vi "ATE_NS_DL_cal2.vi"() -> ()   [LabVIEW 2009]
doc: "Use this template to build a producer/consumer design pattern with events to produce queue items. Use this design pattern instead of the User Interface Event Handler pattern for user interfaces when you want to execute code asynchronously in response to an event without slowing the user interface responsiveness."
uses:
  Rvp8PowerData.ctl
  <vilib>/Analysis/NI_AALBase.lvlib
panel:
  in  "70 dB Attn":i32=70 min=0 max=70 step=10
  in  "READY":bool
  out "Instructions":string="Noise Source Dummy Load calibration vi\n\n1 - Disable or turn off transmitter\n2 - Stow Antenna (point vertically)\n3 - Turn off all florescnt lights\n3 - Start the labview program by clicking the Run arrow\n     (left most button under  drop down menues)\n     start cycle time about 35 seconds\n4 - Wait for the red 'BUSY' light to change to green 'READY'\n     All the control buttons on the control panel are avtive.\n5 - Calibrate with the red  'Calibrate' button\n      calibration cycle time is about ? minutes\n6 - Exit the program with the red 'EXIT' button\n      exit cycle time about 20 seconds\n\nHints:\nWait for the green 'READY' light before clicking buttons\nAll the status leds on the 'Status' tab should be green during a calibration. "
  in  "Configuration 1":bool
  out "Cal Output File":path
  out "Cal file name":string
  in  "Cal data directory":string="/home/operator/ate/data/rvp8_cal"
  in  "Set SigGen":bool
  in  "Initialize":bool
  in  "70 dB":bool
  in  "121 dB":bool
  in  "Switches":bool
  in  "Calibrate":bool
  in  "Stop":bool
  in  "ATE TABS":enum32{"Status", "Controls"}(tab)=enum."Controls"
  out "ATE Switch Status":T1
  out "RVP8 Power":T2 {"time" format="%<%H:%M:%S\n%Y/%m/%d>T"}
  out "121dB\nAttenuators":bool[](array[boolean])
  out "121 Verified":bool
  out "Inside Noise Box":bool
  in  "WG3 MS":bool
  in  "WG3 T":bool
  out "WG3":bool
  in  "WG2 MS":bool
  in  "WG2 T":bool
  out "WG2":bool
  in  "WG1 MS":bool
  in  "WG1 T":bool
  out "WG1":bool
  in  "WG5 ANT":bool
  in  "WG5 DL":bool
  out "WG5":bool
  in  "WG4 ANT":bool
  in  "WG4 DL":bool
  out "WG4":bool
  in  "ATE Switches":T3={"Reversing Switch"=enum."Normal Function", "IO Switch #1 Input"=enum."NONE", "IO Switch #1 Output"=enum."NONE", "IO Switch #2 Input"=enum."NONE", "IO Switch #2 Output"=enum."NONE", "Signal Out Input"=enum."NONE", "Signal Out Output"=enum."NONE", "Signal Source Input"=enum."NONE", "Signal Source Output"=enum."NONE", "Power Meter Switch Input"=enum."NONE", "Pouer Meter Switch Output"=enum."NONE", "Amplifier Switch"=enum."Include Amp"}
  in  "DataSource":bool=TRUE
  in  "Measurements":i32=10
  in  "121 dB Atten":i32 min=0 max=121 step=1
  in  "NoiseSource":bool
  in  "NS_on/off":bool
  in  "Wave Guide Termination":bool
  out "P-State":string
  out "C-State":string
  in  "BUSY":bool
  # "ATE NS DL Program"
  # "1 dB"
  # "2 dB"
  # "4 dB"
  # "4 dB"
  # "10 dB"
  # "20 dB"
  # "40 dB"
  # "40 dB"
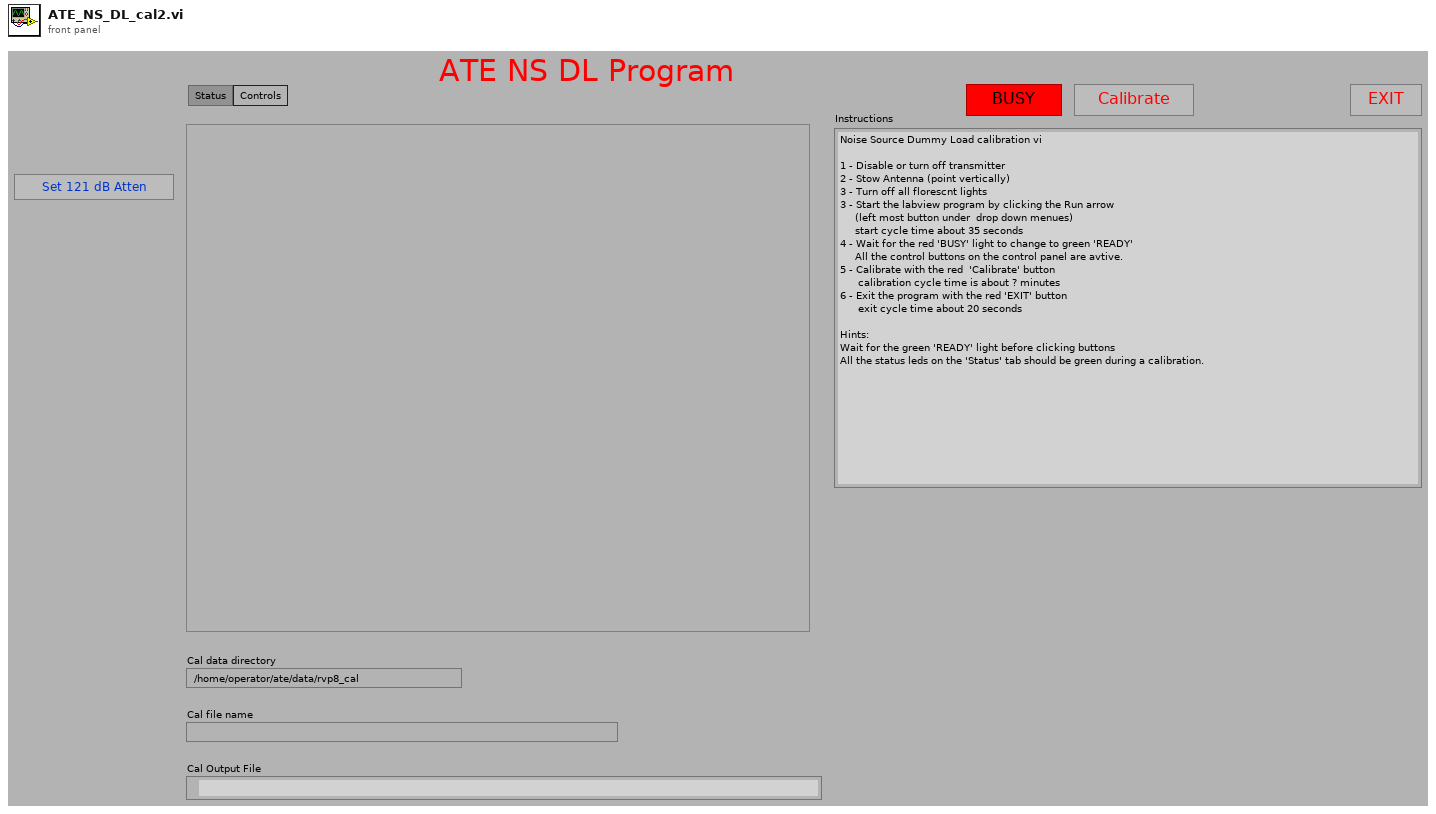
[diagram p1: front panel]
types:
  T1 = cluster{"Reversing Switch ":bool, "IO Switch #1":bool, "IO Switch #2":bool, "Signal Out":bool, "Signal Source":bool, "Power Meter":bool, "Amp By Pass":bool}
  T2 = typedef "Rvp8PowerData.ctl" = cluster{"success":bool, "time":dbl, "el":dbl, "az":dbl, "dbm0":dbl, "dbm1":dbl, "dbmHc":dbl, "dbmHx":dbl, "dbmVc":dbl, "dbmVx":dbl}
  T3 = cluster{"Reversing Switch":enum16{"Normal Function", "Reversing Function"}, "IO Switch #1 Input":enum16{"NONE", "AHR (J2)", "Splitter", "Signal Out Switch (S3)", "Reversing Switch"}, "IO Switch #1 Output":enum16{"NONE", "AHR (J2)", "Delay Device (S4)", "Power Meter Switch (S5)", "Reversing Switch"}, "IO Switch #2 Input":enum16{"NONE", "AVR (J3)", "Splitter", "Signal Out Switch (S3)", " 2W Term (TM1)", "Reversing Switch"}, "IO Switch #2 Output":enum16{"NONE", "AVR (J3)", "Signal Out Switch (S3)", "Power Meter Switch (S5)", "Reversing Switch", "2W Term (TM1)"}, "Signal Out Input":enum16{"NONE", "Amp Bypass Switch (S6)", "IO Switch #1 (S1)", "IO Switch #2 (S2)", "2W Term (TM3)"}, "Signal Out Output":enum16{"NONE", "2 Watt Term (TM3)", "Splitter", "Power Meter Switch (S5)"}, "Signal Source Input":enum16{"NONE", "Delay Device", "Signal Generator (J7)", "Inside Noise Box NF (J5)", "2W Term (TM3)"}, "Signal Source Output":enum16{"NONE", "Amp Bypass Switch", "Test Pulse Generator", "Power Meter Switch (S5)"}, "Power Meter Switch Input":enum16{"NONE", "IO Switch #1 (S1)", "Signal Source Switch (S4)", "Signal Out Switch (S3)", "IO Switch #2 (S2)", "TXH-TXV Switch (J8)"}, "Pouer Meter Switch Output":enum16{"NONE", "Power Meter (J6)"}, "Amplifier Switch":enum16{"Bypass Amp", "Include Amp"}}
  T4 = cluster{"Frequency (GHz)":dbl, "RF Power (dBm)":dbl, "RF ON/OFF":bool}
  T5 = enum16{"open", "replace", "create", "open or create", "replace or create", "replace or create with confirmation"}
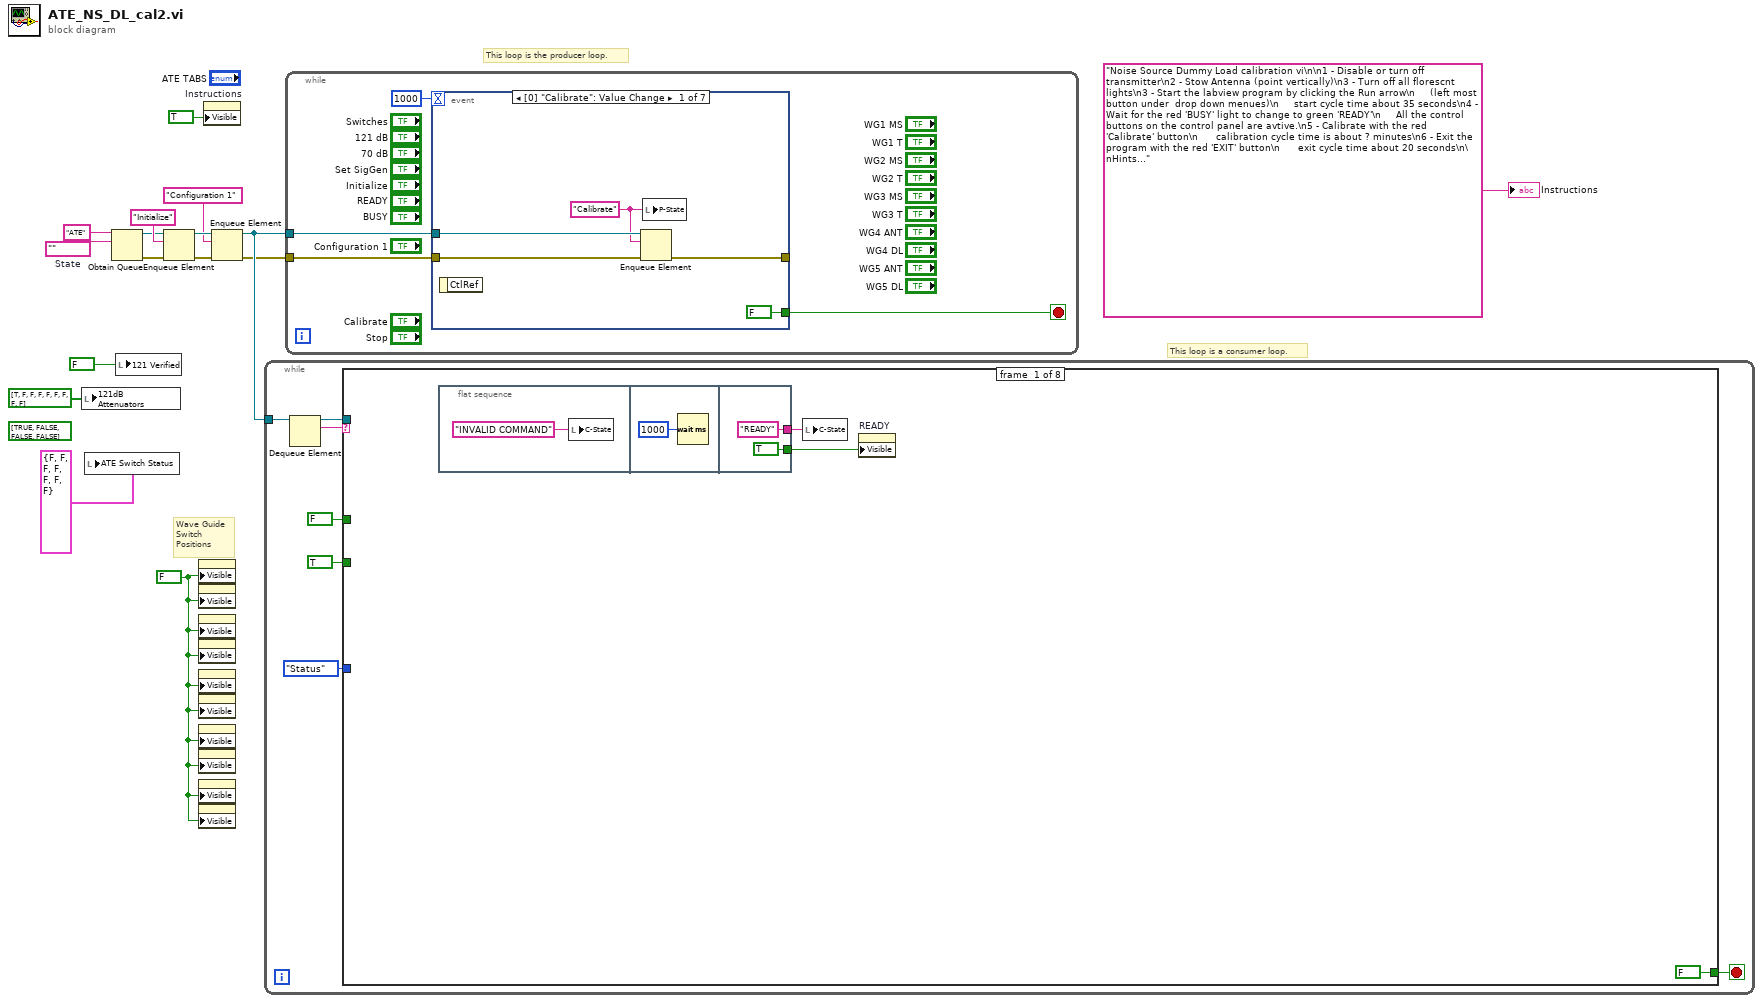
[diagram p0: block diagram]
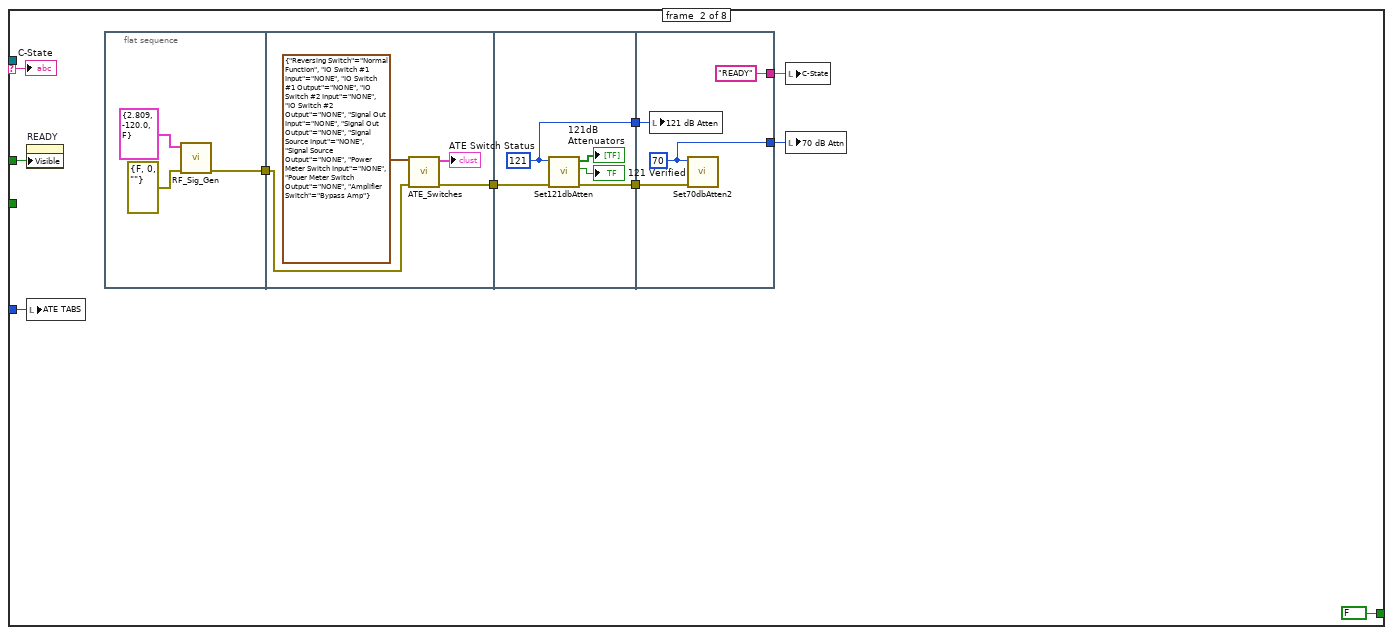
[diagram p2: hidden frame]
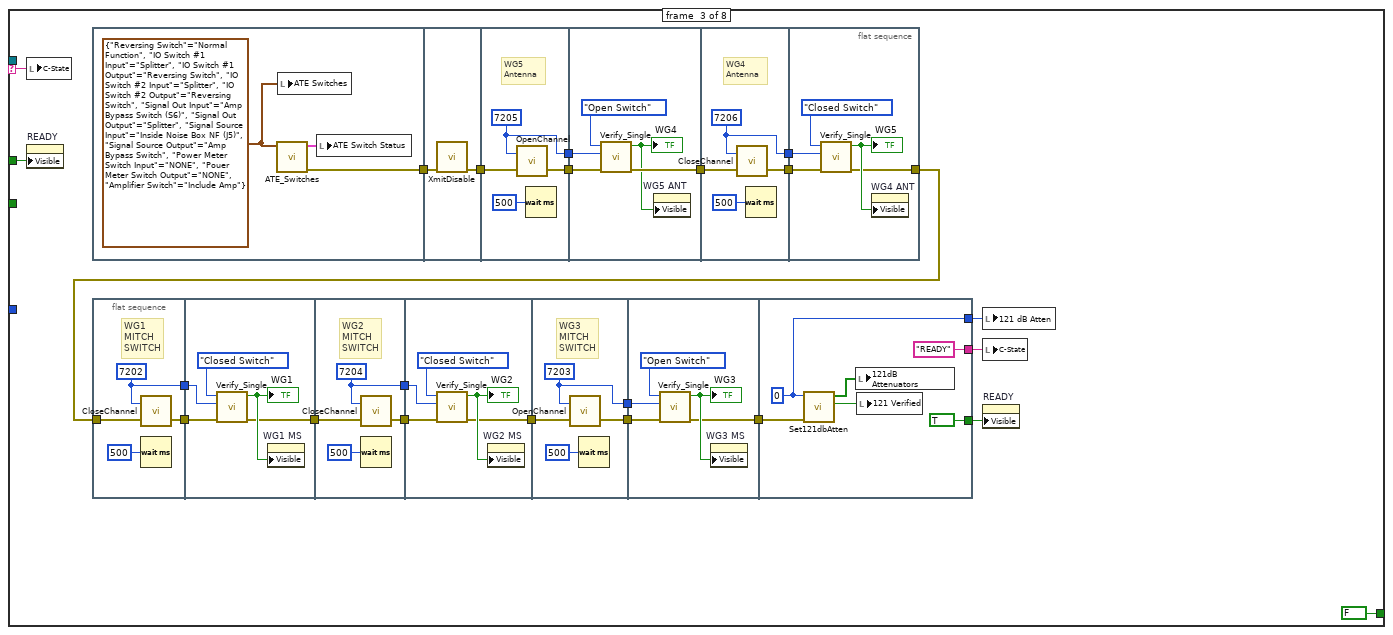
[diagram p3: hidden frame]
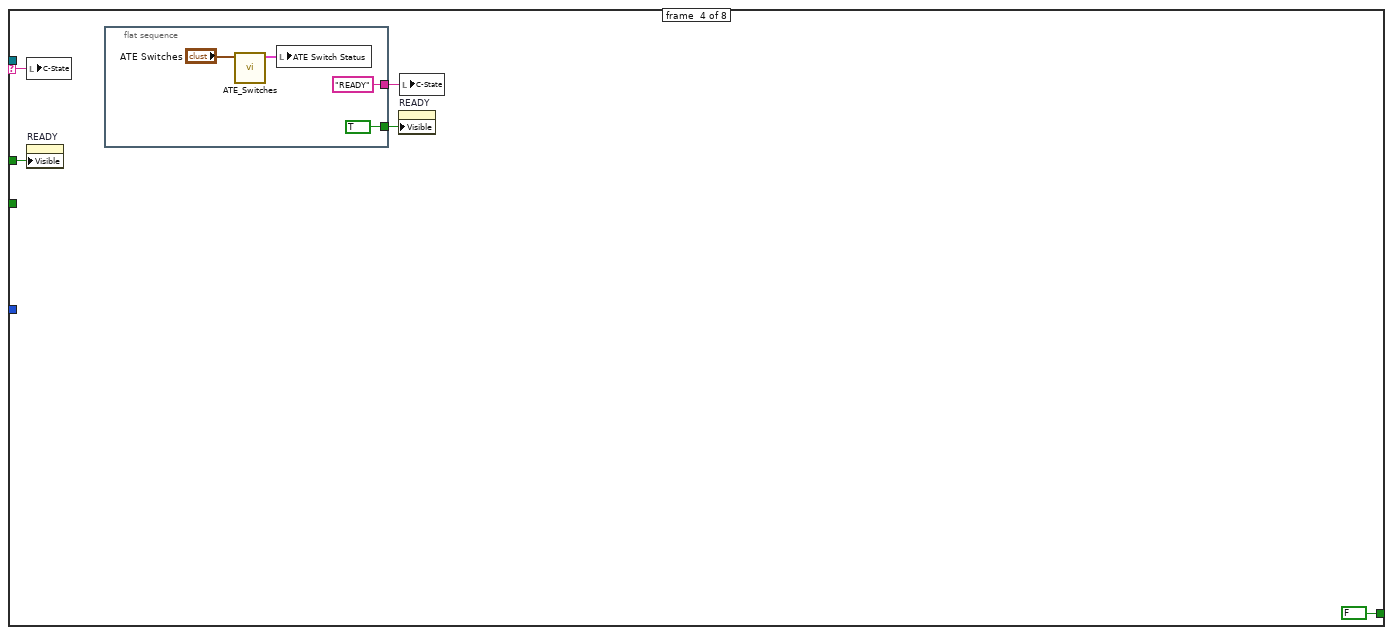
[diagram p4: hidden frame]
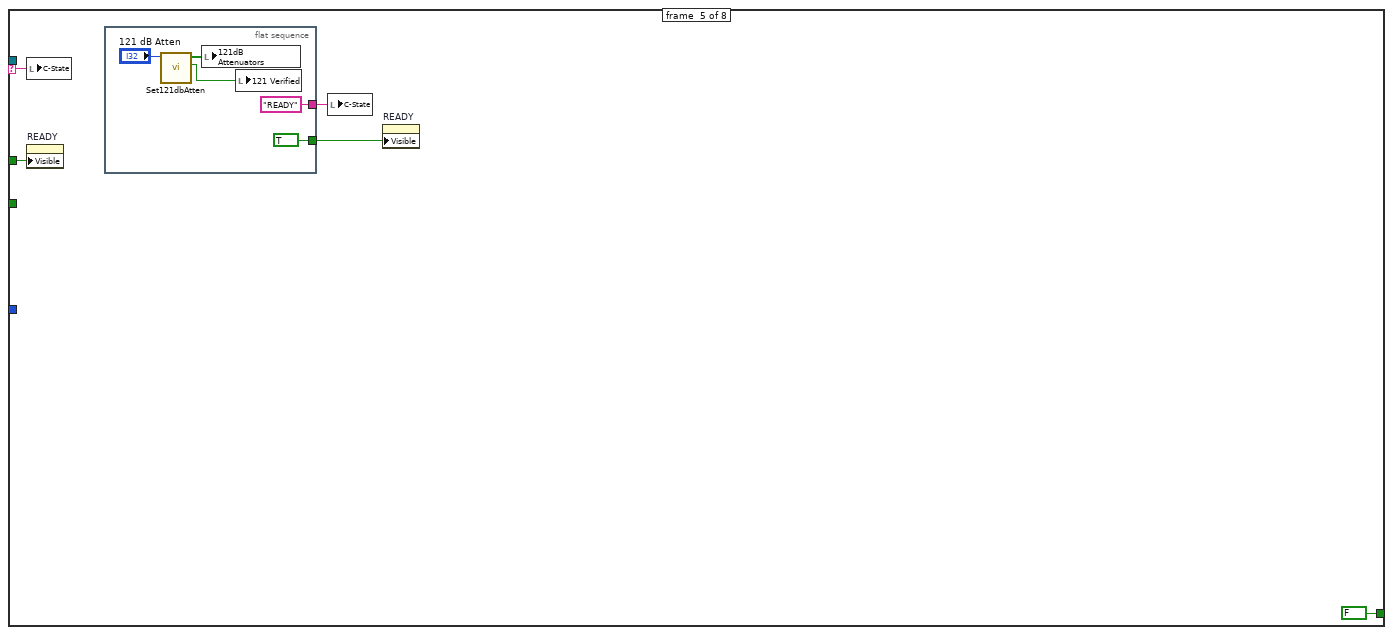
[diagram p5: hidden frame]
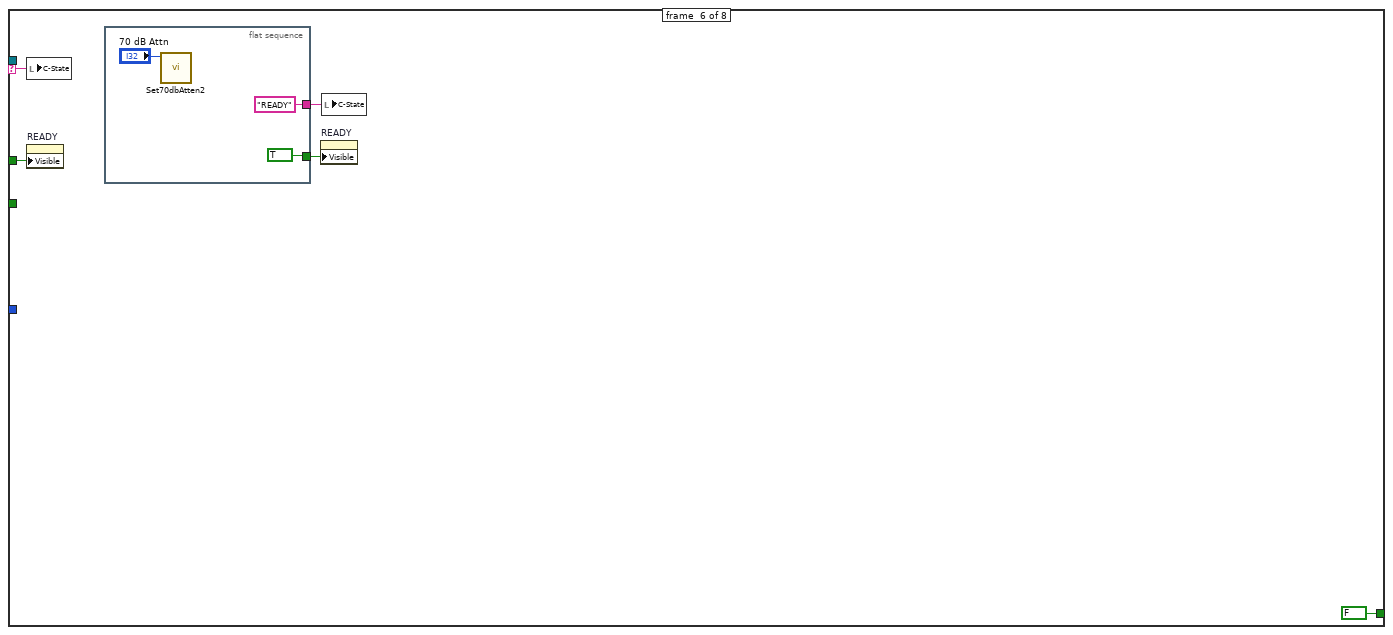
[diagram p6: hidden frame]
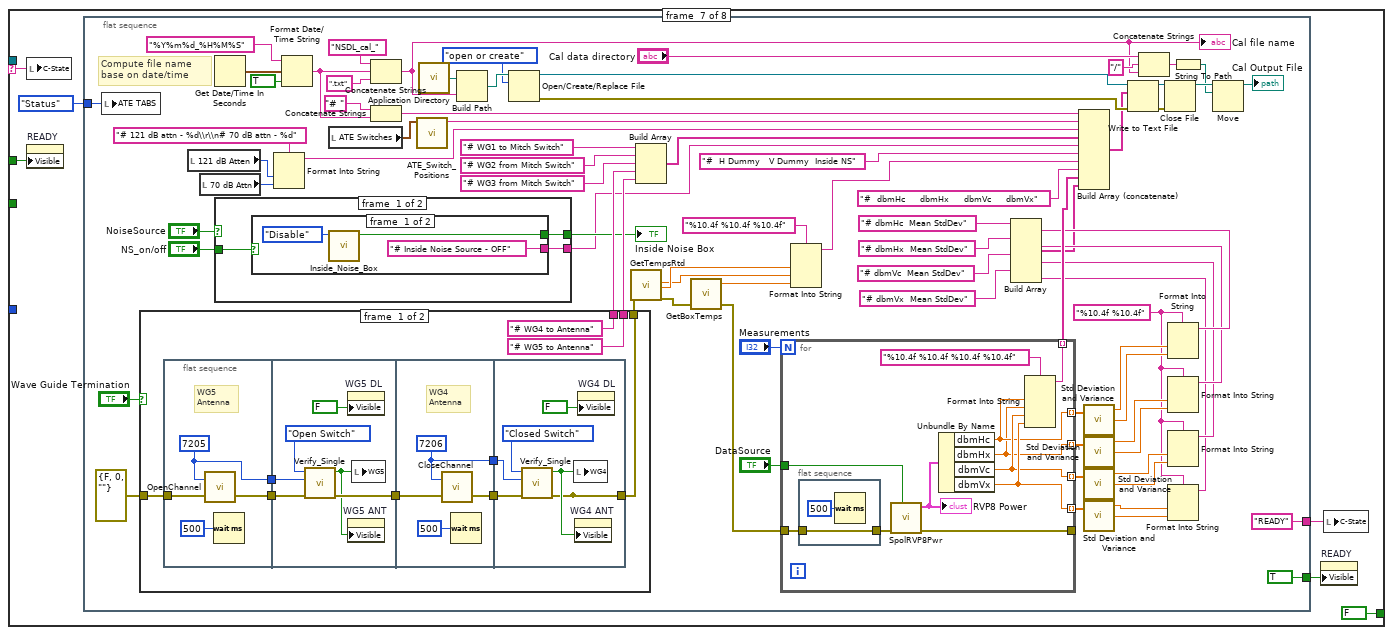
[diagram p7: hidden frame]
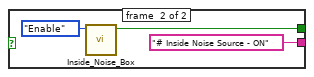
[diagram p8: hidden frame]
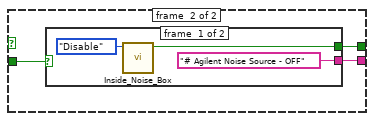
[diagram p9: hidden frame]
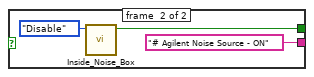
[diagram p10: hidden frame]
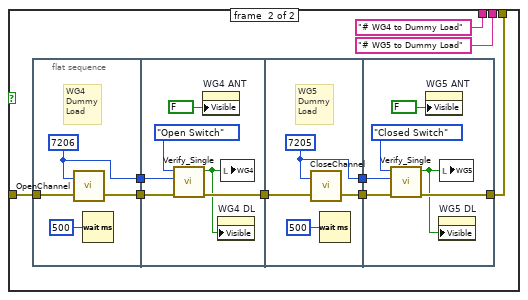
[diagram p11: hidden frame]
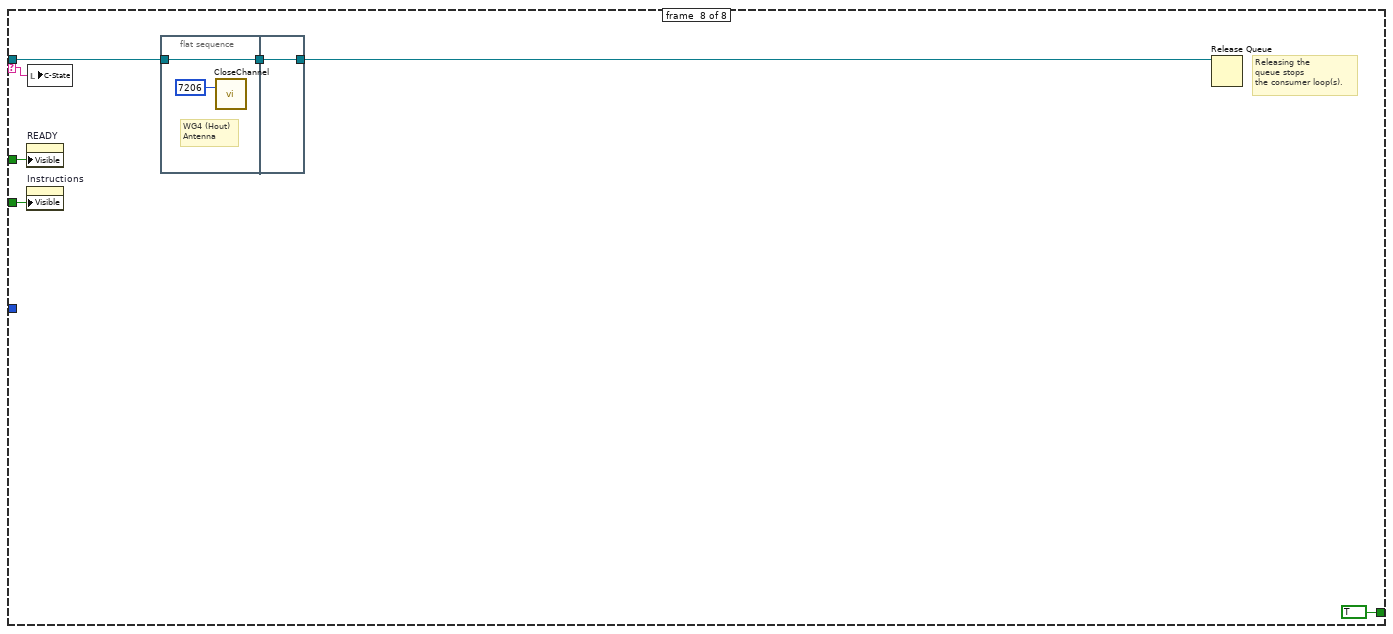
[diagram p12: hidden frame]
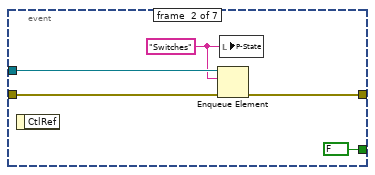
[diagram p13: hidden frame]
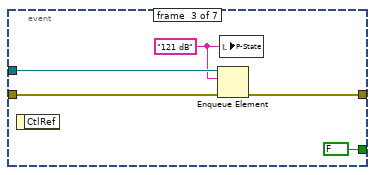
[diagram p14: hidden frame]
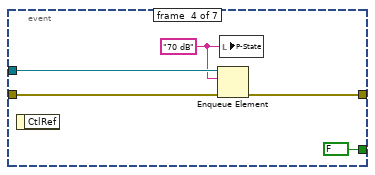
[diagram p15: hidden frame]
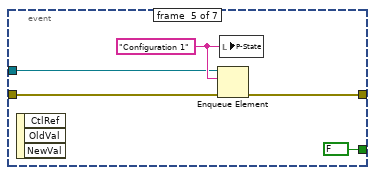
[diagram p16: hidden frame]
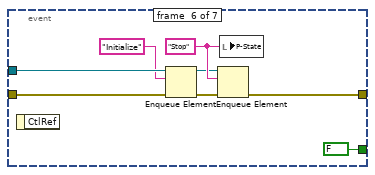
[diagram p17: hidden frame]
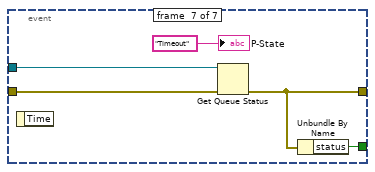
[diagram p18: hidden frame]
diagram:
  w5 = FALSE ("Visible")
  (unwired) bool[] [TRUE, FALSE, FALSE, FALSE] ("70dB\nAttenuators")
  w16 = ""  # State
  # "Wave Guide\nSwitch\nPositions"
  # "This loop is the producer loop."
  # "This loop is a consumer loop."
  n1 = local write "121dB\nAttenuators"(bool[] [TRUE, FALSE, FALSE, FALSE, FALSE, FALSE, FALSE, FALSE, FALSE] ("121dB\nAttenuators")) -> ()
  n2 = local write "ATE Switch Status"(T1 {"Reversing Switch "=FALSE, "IO Switch #1"=FALSE, "IO Switch #2"=FALSE, "Signal Out"=FALSE, "Signal Source"=FALSE, "Power Meter"=FALSE, "Amp By Pass"=FALSE} ("ATE Switch Status")) -> ()
  n3 = Obtain Queue(name (unnamed)="ATE", element data type=w16) -> (queue out=w13:refnum<queue>, error out=w12:errorcluster)  [unwired: 3 in, 1 out]
  n4 = local write "121 Verified"(FALSE ("70 Verfied")) -> ()
  n5 = Enqueue Element(queue=w13, element="Initialize", error in (no error)=w12) -> (queue out=w6:refnum<queue>, error out=w3:errorcluster)  [unwired: 1 in, 1 out]
  n6 = property on="WG1 MS" class="Bool"("Visible"=w5) -> ()  [unwired: 2 in, 2 out]
  n7 = property on="WG1 T" class="Bool"("Visible"=w5) -> ()  [unwired: 2 in, 2 out]
  n8 = property on="WG2 MS" class="Bool"("Visible"=w5) -> ()  [unwired: 2 in, 2 out]
  n9 = property on="WG2 T" class="Bool"("Visible"=w5) -> ()  [unwired: 2 in, 2 out]
  n10 = property on="WG3 MS" class="Bool"("Visible"=w5) -> ()  [unwired: 2 in, 2 out]
  n11 = property on="WG3 T" class="Bool"("Visible"=w5) -> ()  [unwired: 2 in, 2 out]
  n12 = property on="WG4 ANT" class="Bool"("Visible"=w5) -> ()  [unwired: 2 in, 2 out]
  n13 = property on="WG4 DL" class="Bool"("Visible"=w5) -> ()  [unwired: 2 in, 2 out]
  n14 = property on="WG5 ANT" class="Bool"("Visible"=w5) -> ()  [unwired: 2 in, 2 out]
  n15 = property on="WG5 DL" class="Bool"("Visible"=w5) -> ()  [unwired: 2 in, 2 out]
  n16 = property on="Instructions" class="Str"("Visible"=TRUE) -> ()  [unwired: 2 in, 2 out]
  n17 = Enqueue Element(queue=w6, element="Configuration 1", error in (no error)=w3) -> (queue out=w4:refnum<queue>, error out=w2:errorcluster)  [unwired: 1 in, 1 out]
  n18 = while {
    tunnel: w4 -> [w23]
    stop <- w20 stop-if-true
    n19 = Dequeue Element(queue=w23) -> (queue out=w21:refnum<queue>, element=w22:string)  [unwired: 2 in, 2 out]
    n20 = case shown="\"Calibrate\"" w22 {
      selector: w22 -> [_ w39 w77 w140 w148 w158 w167 w342]
      tunnel: w21 -> [_ _ _ _ _ _ _ w339]
      tunnel: [FALSE FALSE FALSE FALSE FALSE FALSE FALSE TRUE] -> w20
      tunnel: FALSE ("Visible") -> [_ w32 w76 w137 w146 w156 w165 w341]
      tunnel: TRUE ("Visible") -> [_ _ _ _ _ _ _ w340]
      tunnel: enum32{"Status", "Controls"}."Status" ("ATE TABS") -> [_ w31 _ _ _ _ _ _]
      frame #0 {
        n21 = flat-sequence {
          tunnel: ["READY" ("element")] -> w25
          tunnel: [TRUE ("Visible")] -> w24
          frame #0 {
            n22 = local write "C-State"("INVALID COMMAND" ("C-State")) -> ()
          }
          frame #1 {
            n23 = Wait (ms)(milliseconds to wait=u32 1000) -> ()  [unwired: 1 out]
          }
          frame #2 {
          }
        }
        n24 = local write "C-State"(w25) -> ()
        n25 = property on="READY" class="Bool"("Visible"=w24) -> ()  [unwired: 2 in, 2 out]
      }
      frame #1 {
        n26 = property on="READY" class="Bool"("Visible"=w32) -> ()  [unwired: 2 in, 2 out]
        n27 = local write "ATE TABS"(w31) -> ()
        n28 = flat-sequence {
          tunnel: [w41] -> w33
          tunnel: [w45] -> w36
          tunnel: w33 -> [w46]
          tunnel: w36 -> [w51]
          tunnel: [w50] -> w37
          tunnel: [w49] -> w35
          tunnel: ["READY" ("element")] -> w38
          tunnel: w37 -> [w56]
          tunnel: w35 -> [w54]
          tunnel: [w53] -> w34
          frame #0 {
            n29 = call "RF_Sig_Gen.vi"("error in"=errorcluster {"status"=FALSE, "code"=0, "source"=""}, "Signal Generator Control"=T4 {"Frequency (GHz)"=2.809, "RF Power (dBm)"=-120.0, "RF ON/OFF"=FALSE}) -> ("Sig Gen Errors"=w41:errorcluster)  [unwired: 8 in, 1 out]
          }
          frame #1 {
            n30 = call "ATE_Switches.vi"("error in"=w46, "ATE Switches"=T3 {"Reversing Switch"=enum."Normal Function", "IO Switch #1 Input"=enum."NONE", "IO Switch #1 Output"=enum."NONE", "IO Switch #2 Input"=enum."NONE", "IO Switch #2 Output"=enum."NONE", "Signal Out Input"=enum."NONE", "Signal Out Output"=enum."NONE", "Signal Source Input"=enum."NONE", "Signal Source Output"=enum."NONE", "Power Meter Switch Input"=enum."NONE", "Pouer Meter Switch Output"=enum."NONE", "Amplifier Switch"=enum."Bypass Amp"}) -> ("Switch Errors"=w45:errorcluster, "ATE Switch Status"=→"ATE Switch Status":T1)  [unwired: 8 in]
          }
          frame #2 {
            w49 = 121 ("Attenuation (dB)")
            n31 = call "Set121dbAtten.vi"("error in (no error)"=w51, "Attenuation (dB)"=w49) -> ("error out"=w50:errorcluster, "Verfied"=→"121 Verified":bool, "Active Attenuators"=→"121dB\nAttenuators":bool[])  [unwired: 7 in]
          }
          frame #3 {
            w53 = 70 ("Attenuation (dB)")
            n32 = local write "121 dB Atten"(w54) -> ()
            n33 = call "Set70dbAtten2.vi"("error in (no error)"=w56, "Attenuation (dB)"=w53) -> ()  [unwired: 7 in, 3 out]
          }
        }
        n34 = local write "C-State"(w38) -> ()
        n35 = local write "70 dB Attn"(w34) -> ()
        "C-State" <- w39
      }
      frame #2 {
        n36 = local write "C-State"(w77) -> ()
        n37 = property on="READY" class="Bool"("Visible"=w76) -> ()  [unwired: 2 in, 2 out]
        n38 = flat-sequence {
          tunnel: [w115] -> w78
          tunnel: w78 -> [w117]
          tunnel: [w116] -> w75
          tunnel: w75 -> [w121]
          tunnel: [w120] -> w72
          tunnel: [w119] -> w71
          tunnel: [w123] -> w74
          tunnel: w72 -> [w125]
          tunnel: w71 -> [w124]
          tunnel: [w128] -> w73
          tunnel: w74 -> [w130]
          tunnel: [w127] -> w59
          tunnel: w73 -> [w134]
          tunnel: w59 -> [w133]
          tunnel: [w131] -> w58
          frame #0 {
            w113 = T3 {"Reversing Switch"=enum."Normal Function", "IO Switch #1 Input"=enum."Splitter", "IO Switch #1 Output"=enum."Reversing Switch", "IO Switch #2 Input"=enum."Splitter", "IO Switch #2 Output"=enum."Reversing Switch", "Signal Out Input"=enum."Amp Bypass Switch (S6)", "Signal Out Output"=enum."Splitter", "Signal Source Input"=enum."Inside Noise Box NF (J5)", "Signal Source Output"=enum."Amp Bypass Switch", "Power Meter Switch Input"=enum."NONE", "Pouer Meter Switch Output"=enum."NONE", "Amplifier Switch"=enum."Include Amp"} ("ATE Switches")
            n39 = call "ATE_Switches.vi"("ATE Switches"=w113) -> ("Switch Errors"=w115:errorcluster, "ATE Switch Status"=w114:T1)  [unwired: 9 in]
            n40 = local write "ATE Switches"(w113) -> ()
            n41 = local write "ATE Switch Status"(w114) -> ()
          }
          frame #1 {
            n42 = call "XmitDisable.vi"("error in (no error)"=w117) -> ("error out"=w116:errorcluster)  [unwired: 1 in, 5 out]
          }
          frame #2 {
            w119 = 7205
            # "WG5\nAntenna"
            n43 = call "OpenChannel.vi"("error in (no error)"=w121, "Channel ID"=w119) -> ("error out"=w120:errorcluster)  [unwired: 1 in]
            n44 = Wait (ms)(milliseconds to wait=u32 500) -> ()  [unwired: 1 out]
          }
          frame #3 {
            n45 = call "Verify_Single.vi"("error in"=w125, "Switch ID"=w124, "Switch Functin"=enum16{"Open Switch", "Closed Switch"}."Open Switch") -> ("Error out"=w123:errorcluster, "Verfied"=w122:bool)  [unwired: 7 in]
            "WG4" <- w122
            n46 = property on="WG5 ANT" class="Bool"("Visible"=w122) -> ()  [unwired: 2 in, 2 out]
          }
          frame #4 {
            w127 = 7206
            # "WG4\nAntenna"
            n47 = call "CloseChannel.vi"("error in (no error)"=w130, "Channel ID"=w127) -> ("error out"=w128:errorcluster)  [unwired: 1 in]
            n48 = Wait (ms)(milliseconds to wait=u32 500) -> ()  [unwired: 1 out]
          }
          frame #5 {
            n49 = call "Verify_Single.vi"("error in"=w134, "Switch ID"=w133, "Switch Functin"=enum16{"Open Switch", "Closed Switch"}."Closed Switch") -> ("Error out"=w131:errorcluster, "Verfied"=w132:bool)  [unwired: 7 in]
            "WG5" <- w132
            n50 = property on="WG4 ANT" class="Bool"("Visible"=w132) -> ()  [unwired: 2 in, 2 out]
          }
        }
        n51 = flat-sequence {
          tunnel: [w82] -> w70
          tunnel: [w81] -> w67
          tunnel: w58 -> [w80]
          tunnel: w70 -> [w87]
          tunnel: [w85] -> w69
          tunnel: w67 -> [w84]
          tunnel: w69 -> [w91]
          tunnel: [w90] -> w68
          tunnel: [w89] -> w66
          tunnel: w68 -> [w96]
          tunnel: w66 -> [w95]
          tunnel: [w93] -> w65
          tunnel: w65 -> [w100]
          tunnel: [w99] -> w64
          tunnel: [w98] -> w63
          tunnel: w64 -> [w104]
          tunnel: w63 -> [w105]
          tunnel: [w102] -> w62
          tunnel: w62 -> [w108]
          tunnel: [TRUE ("Visible")] -> w61
          tunnel: ["READY" ("element")] -> w60
          tunnel: [w107] -> w57
          frame #0 {
            w81 = 7202
            # "WG1\nMITCH\nSWITCH"
            n52 = call "CloseChannel.vi"("error in (no error)"=w80, "Channel ID"=w81) -> ("error out"=w82:errorcluster)  [unwired: 1 in]
            n53 = Wait (ms)(milliseconds to wait=u32 500) -> ()  [unwired: 1 out]
          }
          frame #1 {
            n54 = call "Verify_Single.vi"("error in"=w87, "Switch ID"=w84, "Switch Functin"=enum16{"Open Switch", "Closed Switch"}."Closed Switch") -> ("Error out"=w85:errorcluster, "Verfied"=w86:bool)  [unwired: 7 in]
            "WG1" <- w86
            n55 = property on="WG1 MS" class="Bool"("Visible"=w86) -> ()  [unwired: 2 in, 2 out]
          }
          frame #2 {
            w89 = 7204
            # "WG2\nMITCH\nSWITCH"
            n56 = call "CloseChannel.vi"("error in (no error)"=w91, "Channel ID"=w89) -> ("error out"=w90:errorcluster)  [unwired: 1 in]
            n57 = Wait (ms)(milliseconds to wait=u32 500) -> ()  [unwired: 1 out]
          }
          frame #3 {
            n58 = call "Verify_Single.vi"("error in"=w96, "Switch ID"=w95, "Switch Functin"=enum16{"Open Switch", "Closed Switch"}."Closed Switch") -> ("Error out"=w93:errorcluster, "Verfied"=w94:bool)  [unwired: 7 in]
            "WG2" <- w94
            n59 = property on="WG2 MS" class="Bool"("Visible"=w94) -> ()  [unwired: 2 in, 2 out]
          }
          frame #4 {
            w99 = 7203
            # "WG3\nMITCH\nSWITCH"
            n60 = call "OpenChannel.vi"("error in (no error)"=w100, "Channel ID"=w99) -> ("error out"=w98:errorcluster)  [unwired: 1 in]
            n61 = Wait (ms)(milliseconds to wait=u32 500) -> ()  [unwired: 1 out]
          }
          frame #5 {
            n62 = call "Verify_Single.vi"("error in"=w105, "Switch ID"=w104, "Switch Functin"=enum16{"Open Switch", "Closed Switch"}."Open Switch") -> ("Error out"=w102:errorcluster, "Verfied"=w103:bool)  [unwired: 7 in]
            "WG3" <- w103
            n63 = property on="WG3 MS" class="Bool"("Visible"=w103) -> ()  [unwired: 2 in, 2 out]
          }
          frame #6 {
            w107 = 0 ("Attenuation (dB)")
            n64 = call "Set121dbAtten.vi"("error in (no error)"=w108, "Attenuation (dB)"=w107) -> ("Verfied"=w109:bool, "Active Attenuators"=w110:bool[])  [unwired: 7 in, 1 out]
            n65 = local write "121dB\nAttenuators"(w110) -> ()
            n66 = local write "121 Verified"(w109) -> ()
          }
        }
        n67 = local write "121 dB Atten"(w57) -> ()
        n68 = local write "C-State"(w60) -> ()
        n69 = property on="READY" class="Bool"("Visible"=w61) -> ()  [unwired: 2 in, 2 out]
      }
      frame #3 {
        n70 = local write "C-State"(w140) -> ()
        n71 = property on="READY" class="Bool"("Visible"=w137) -> ()  [unwired: 2 in, 2 out]
        n72 = flat-sequence {
          tunnel: ["READY" ("element")] -> w138
          tunnel: [TRUE ("Visible")] -> w136
          frame #0 {
            n73 = call "ATE_Switches.vi"("ATE Switches"="ATE Switches") -> ("ATE Switch Status"=w143:T1)  [unwired: 9 in, 1 out]
            n74 = local write "ATE Switch Status"(w143) -> ()
          }
        }
        n75 = property on="READY" class="Bool"("Visible"=w136) -> ()  [unwired: 2 in, 2 out]
        n76 = local write "C-State"(w138) -> ()
      }
      frame #4 {
        n77 = local write "C-State"(w148) -> ()
        n78 = property on="READY" class="Bool"("Visible"=w146) -> ()  [unwired: 2 in, 2 out]
        n79 = flat-sequence {
          tunnel: ["READY" ("element")] -> w147
          tunnel: [TRUE ("Visible")] -> w145
          frame #0 {
            n80 = call "Set121dbAtten.vi"("Attenuation (dB)"="121 dB Atten") -> ("Verfied"=w151:bool, "Active Attenuators"=w153:bool[])  [unwired: 8 in, 1 out]
            n81 = local write "121dB\nAttenuators"(w153) -> ()
            n82 = local write "121 Verified"(w151) -> ()
          }
        }
        n83 = local write "C-State"(w147) -> ()
        n84 = property on="READY" class="Bool"("Visible"=w145) -> ()  [unwired: 2 in, 2 out]
      }
      frame #5 {
        n85 = local write "C-State"(w158) -> ()
        n86 = property on="READY" class="Bool"("Visible"=w156) -> ()  [unwired: 2 in, 2 out]
        n87 = flat-sequence {
          tunnel: ["READY" ("element")] -> w157
          tunnel: [TRUE ("Visible")] -> w155
          frame #0 {
            n88 = call "Set70dbAtten2.vi"("Attenuation (dB)"="70 dB Attn") -> ()  [unwired: 8 in, 3 out]
          }
        }
        n89 = property on="READY" class="Bool"("Visible"=w155) -> ()  [unwired: 2 in, 2 out]
        n90 = local write "C-State"(w157) -> ()
      }
      frame #6 {
        n91 = local write "C-State"(w167) -> ()
        n92 = property on="READY" class="Bool"("Visible"=w165) -> ()  [unwired: 2 in, 2 out]
        n93 = flat-sequence {
          tunnel: ["READY" ("element")] -> w166
          tunnel: [TRUE ("Visible")] -> w164
          tunnel: enum32{"Status", "Controls"}."Status" ("ATE TABS") -> [w215]
          frame #0 {
            w169 = "%10.4f %10.4f"
            # "Compute file name base on date/time"
            n94 = local write "ATE TABS"(w215) -> ()
            n95 = case shown="True" "Wave Guide Termination" {
              tunnel: errorcluster {"status"=FALSE, "code"=0, "source"=""} ("error out") -> [w269 w298]
              tunnel: [w268 w297] -> w201
              tunnel: ["# WG4 to Antenna" "# WG4 to Dummy Load"] -> w209
              tunnel: ["# WG5 to Antenna" "# WG5 to Dummy Load"] -> w208
              frame #0 {
                n96 = flat-sequence {
                  tunnel: [w277] -> w274
                  tunnel: [w276] -> w273
                  tunnel: w269 -> [w275]
                  tunnel: w274 -> [w283]
                  tunnel: [w282] -> w272
                  tunnel: w273 -> [w281]
                  tunnel: w272 -> [w287]
                  tunnel: [w286] -> w271
                  tunnel: [w285] -> w270
                  tunnel: w271 -> [w293]
                  tunnel: [w289] -> _
                  tunnel: w270 -> [w292]
                  tunnel: [w289] -> w268
                  frame #0 {
                    w276 = 7205
                    # "WG5\nAntenna"
                    n97 = call "OpenChannel.vi"("error in (no error)"=w275, "Channel ID"=w276) -> ("error out"=w277:errorcluster)  [unwired: 1 in]
                    n98 = Wait (ms)(milliseconds to wait=u32 500) -> ()  [unwired: 1 out]
                  }
                  frame #1 {
                    n99 = call "Verify_Single.vi"("error in"=w283, "Switch ID"=w281, "Switch Functin"=enum16{"Open Switch", "Closed Switch"}."Open Switch") -> ("Error out"=w282:errorcluster, "Verfied"=w280:bool)  [unwired: 7 in]
                    n100 = property on="WG5 DL" class="Bool"("Visible"=FALSE) -> ()  [unwired: 2 in, 2 out]
                    n101 = property on="WG5 ANT" class="Bool"("Visible"=w280) -> ()  [unwired: 2 in, 2 out]
                    n102 = local write "WG5"(w280) -> ()
                  }
                  frame #2 {
                    w285 = 7206
                    # "WG4\nAntenna"
                    n103 = call "CloseChannel.vi"("error in (no error)"=w287, "Channel ID"=w285) -> ("error out"=w286:errorcluster)  [unwired: 1 in]
                    n104 = Wait (ms)(milliseconds to wait=u32 500) -> ()  [unwired: 1 out]
                  }
                  frame #3 {
                    n105 = call "Verify_Single.vi"("error in"=w293, "Switch ID"=w292, "Switch Functin"=enum16{"Open Switch", "Closed Switch"}."Closed Switch") -> ("Error out"=w289:errorcluster, "Verfied"=w291:bool)  [unwired: 7 in]
                    n106 = local write "WG4"(w291) -> ()
                    n107 = property on="WG4 ANT" class="Bool"("Visible"=w291) -> ()  [unwired: 2 in, 2 out]
                    n108 = property on="WG4 DL" class="Bool"("Visible"=FALSE) -> ()  [unwired: 2 in, 2 out]
                  }
                }
              }
              frame #1 {
                n109 = flat-sequence {
                  tunnel: [w306] -> w303
                  tunnel: [w305] -> w302
                  tunnel: w298 -> [w304]
                  tunnel: w303 -> [w312]
                  tunnel: [w311] -> w301
                  tunnel: w302 -> [w310]
                  tunnel: w301 -> [w316]
                  tunnel: [w315] -> w300
                  tunnel: [w314] -> w299
                  tunnel: w300 -> [w322]
                  tunnel: [w321] -> w297
                  tunnel: w299 -> [w320]
                  frame #0 {
                    w305 = 7206
                    # "WG4\nDummy\nLoad"
                    n110 = call "OpenChannel.vi"("error in (no error)"=w304, "Channel ID"=w305) -> ("error out"=w306:errorcluster)  [unwired: 1 in]
                    n111 = Wait (ms)(milliseconds to wait=u32 500) -> ()  [unwired: 1 out]
                  }
                  frame #1 {
                    n112 = call "Verify_Single.vi"("error in"=w312, "Switch ID"=w310, "Switch Functin"=enum16{"Open Switch", "Closed Switch"}."Open Switch") -> ("Error out"=w311:errorcluster, "Verfied"=w309:bool)  [unwired: 7 in]
                    n113 = property on="WG4 ANT" class="Bool"("Visible"=FALSE) -> ()  [unwired: 2 in, 2 out]
                    n114 = property on="WG4 DL" class="Bool"("Visible"=w309) -> ()  [unwired: 2 in, 2 out]
                    n115 = local write "WG4"(w309) -> ()
                  }
                  frame #2 {
                    w314 = 7205
                    # "WG5\nDummy\nLoad"
                    n116 = call "CloseChannel.vi"("error in (no error)"=w316, "Channel ID"=w314) -> ("error out"=w315:errorcluster)  [unwired: 1 in]
                    n117 = Wait (ms)(milliseconds to wait=u32 500) -> ()  [unwired: 1 out]
                  }
                  frame #3 {
                    n118 = call "Verify_Single.vi"("error in"=w322, "Switch ID"=w320, "Switch Functin"=enum16{"Open Switch", "Closed Switch"}."Closed Switch") -> ("Error out"=w321:errorcluster, "Verfied"=w319:bool)  [unwired: 7 in]
                    n119 = property on="WG5 ANT" class="Bool"("Visible"=FALSE) -> ()  [unwired: 2 in, 2 out]
                    n120 = property on="WG5 DL" class="Bool"("Visible"=w319) -> ()  [unwired: 2 in, 2 out]
                    n121 = local write "WG5"(w319) -> ()
                  }
                }
              }
            }
            n122 = local read "121 dB Atten"() -> (w229:i32)
            n123 = local read "70 dB Attn"() -> (w228:i32)
            n124 = Get Date/Time In Seconds() -> (seconds since 1Jan1904=w242:timestamp)
            n125 = case shown="True" "NoiseSource" {
              tunnel: "NS_on/off" -> [w249 w259]
              tunnel: [w250 w258] -> w170
              tunnel: [w248 w257] -> w204
              frame #0 {
                n126 = case shown="False" w249 {
                  tunnel: ["# Inside Noise Source - OFF" "# Inside Noise Source - ON"] -> w250
                  tunnel: [w251 w254] -> w248
                  frame #0 {
                    n127 = call "Inside_Noise_Box.vi"("Noise Switch Function"=enum16{"Disable", "Enable"}."Disable") -> ("Verfied"=w251:bool)  [unwired: 9 in, 1 out]
                  }
                  frame #1 {
                    n128 = call "Inside_Noise_Box.vi"("Noise Switch Function"=enum16{"Disable", "Enable"}."Enable") -> ("Verfied"=w254:bool)  [unwired: 9 in, 1 out]
                  }
                }
              }
              frame #1 {
                n129 = case shown="True" w259 {
                  tunnel: ["# Agilent Noise Source - OFF" "# Agilent Noise Source - ON"] -> w258
                  tunnel: [w260 w263] -> w257
                  frame #0 {
                    n130 = call "Inside_Noise_Box.vi"("Noise Switch Function"=enum16{"Disable", "Enable"}."Disable") -> ("Verfied"=w260:bool)  [unwired: 9 in, 1 out]
                  }
                  frame #1 {
                    n131 = call "Inside_Noise_Box.vi"("Noise Switch Function"=enum16{"Disable", "Enable"}."Disable") -> ("Verfied"=w263:bool)  [unwired: 9 in, 1 out]
                  }
                }
              }
            }
            "Inside Noise Box" <- w204
            n132 = Format Into String(format string="# 121 dB attn - %d\\r\\n# 70 dB attn - %d", w229, w228) -> (resulting string=w223:string)  [unwired: 2 in, 1 out]
            n133 = Format Date/Time String(time format string (%c)="%Y%m%d_%H%M%S", seconds (now)=w242, UTC format=TRUE) -> (date/time string=w218:string)
            n134 = local read "ATE Switches"() -> (w222:T3)
            n135 = Concatenate Strings("NSDL_cal_", w218, ".txt") -> (w217:string)
            "Cal file name" <- w217
            n136 = Concatenate Strings("# " ("string"), w218) -> (w225:string)
            n137 = call "ATE_Switch_Positions.vi"("ATE Switches"=w222) -> ("ATE Switch/Position"=w224:string)  [unwired: 10 in]
            n138 = call <vilib>:"Application Directory.vi"() -> ("Application Directory"=w219:path)
            n139 = Build Path(base path=w219, name or relative path=w217) -> (appended path=w241:path)
            n140 = Open/Create/Replace File(file path (use dialog)=w241, operation (0:open)=T5."open or create") -> (refnum out=w240:refnum<file>, error out=w239:errorcluster)  [unwired: 4 in, 1 out]
            n141 = call "GetTempsRtd.vi"("error in (no error)"=w201) -> ("Temp V Dummy"=w202:dbl, "Temp H Dummy"=w203:dbl, "error out"=w200:errorcluster)  [unwired: 2 in, 14 out]
            n142 = Build Array("# WG1 to Mitch Switch", "# WG2 from Mitch Switch", "# WG3 from Mitch Switch", w209, w208) -> (w207:string[])
            n143 = call "GetBoxTemps.vi"("error in (no error)"=w200) -> ("error out"=w199:errorcluster, "InsideBox"=w198:dbl)  [unwired: 1 in, 2 out]
            n144 = for {
              N: "Measurements" -> [_]
              tunnel: w199 -> [w328]
              tunnel: [w334] -> w197 mode=indexing
              tunnel: [w329] -> _
              tunnel: "DataSource" -> [w331]
              tunnel: [w327] -> w193 mode=indexing
              tunnel: [w326] -> w190 mode=indexing
              tunnel: [w324] -> w191 mode=indexing
              tunnel: [w325] -> w192 mode=indexing
              n145 = flat-sequence {
                tunnel: w328 -> [w336]
                tunnel: [w336] -> w333
                frame #0 {
                  n146 = Wait (ms)(milliseconds to wait=u32 500) -> ()  [unwired: 1 out]
                }
              }
              n147 = call "SpolRVP8Pwr.vi"("DataSource"=w331, "error in (no error)"=w333) -> ("Comm error"=w329:errorcluster, "RVP8_power"=w330:T2)  [unwired: 6 in, 2 out]
              "RVP8 Power" <- w330
              n148 = Unbundle By Name(w330) -> ("dbmHc"=w325:dbl, "dbmHx"=w324:dbl, "dbmVc"=w326:dbl, "dbmVx"=w327:dbl)
              n149 = Format Into String(format string="%10.4f %10.4f %10.4f %10.4f", w325, w324, w326, w327) -> (resulting string=w334:string)  [unwired: 2 in, 1 out]
            }
            n150 = Format Into String(format string="%10.4f %10.4f %10.4f", w203, w202, w198) -> (resulting string=w189:string)  [unwired: 2 in, 1 out]
            n151 = call <vilib>:"Std Deviation and Variance.vi"("X"=w192) -> ("mean"=w188:dbl, "standard deviation"=w187:dbl)  [unwired: 1 in, 1 out]
            n152 = call <vilib>:"Std Deviation and Variance.vi"("X"=w191) -> ("mean"=w186:dbl, "standard deviation"=w185:dbl)  [unwired: 1 in, 1 out]
            n153 = call <vilib>:"Std Deviation and Variance.vi"("X"=w190) -> ("mean"=w184:dbl, "standard deviation"=w183:dbl)  [unwired: 1 in, 1 out]
            n154 = call <vilib>:"Std Deviation and Variance.vi"("X"=w193) -> ("mean"=w182:dbl, "standard deviation"=w181:dbl)  [unwired: 1 in, 1 out]
            n155 = Concatenate Strings("Cal data directory", "/" ("string"), w217) -> (w235:string)
            n156 = Format Into String(format string=w169, w188, w187) -> (resulting string=w176:string)  [unwired: 2 in, 1 out]
            n157 = Format Into String(format string=w169, w186, w185) -> (resulting string=w175:string)  [unwired: 2 in, 1 out]
            n158 = Format Into String(format string=w169, w184, w183) -> (resulting string=w174:string)  [unwired: 2 in, 1 out]
            n159 = Format Into String(format string=w169, w182, w181) -> (resulting string=w173:string)  [unwired: 2 in, 1 out]
            n160 = Build Array("# dbmHc  Mean StdDev", w176, "# dbmHx  Mean StdDev", w175, "# dbmVc  Mean StdDev", w174, "# dbmVx  Mean StdDev", w173) -> (w172:string[])
            n161 = Build Array (concatenate)(w225, w224, w223, w207, w170, "#  H Dummy   V Dummy  Inside NS", w189, "#  dbmHc     dbmHx     dbmVc     dbmVx", w197, w172) -> (w231:string[])
            n162 = Write to Text File(file (use dialog)=w240, text=w231, error in=w239) -> (refnum out=w238:refnum<file>, error out=w237:errorcluster)  [unwired: 1 in, 1 out]
            n163 = Close File(refnum=w238, error in=w237) -> (path=w234:path)  [unwired: 1 out]
            n164 = String To Path(string=w235) -> (path=w233:path)
            n165 = Move(source path=w234, 10:w233) -> (3:→"Cal Output File":path)  [unwired: 3 in, 2 out]
          }
        }
        n166 = property on="READY" class="Bool"("Visible"=w164) -> ()  [unwired: 2 in, 2 out]
        n167 = local write "C-State"(w166) -> ()
      }
      frame #7 {
        # "Releasing the\nqueue stops\nthe consumer loop(s)."
        n168 = property on="READY" class="Bool"("Visible"=w341) -> ()  [unwired: 2 in, 2 out]
        n169 = property on="Instructions" class="Str"("Visible"=w340) -> ()  [unwired: 2 in, 2 out]
        n170 = local write "C-State"(w342) -> ()
        n171 = flat-sequence {
          tunnel: w339 -> [w345]
          tunnel: [w345] -> w337
          tunnel: [w346] -> w338
          tunnel: w337 -> [w346]
          frame #0 {
            # "WG4 (Hout)\nAntenna"
            n172 = call "CloseChannel.vi"("Channel ID"=7206) -> ()  [unwired: 2 in, 1 out]
          }
          frame #1 {
          }
        }
        n173 = Release Queue(queue=w338) -> ()  [unwired: 2 in, 3 out]
      }
    }
  }
  n174 = while {
    tunnel: w4 -> [w350]
    tunnel: w2 -> [w349]
    stop <- w347 stop-if-true
    n175 = event shown="[0] \"Calibrate\": Value Change" {
      selector: _ -> [_ _ _ _ _ _ _]
      dyn-events: _ -> [_ _ _ _ _ _ _]
      timeout: 1000 -> [_ _ _ _ _ _ _]
      tunnel: w350 -> [w355 w360 w365 w370 w374 w378 w388]
      tunnel: w349 -> [w354 w359 w364 w369 w373 w380 w384]
      tunnel: [w353 w358 w363 w368 w372 w383 w386] -> _
      tunnel: [FALSE FALSE FALSE FALSE FALSE ("status") FALSE w387] -> w347
      event #0 {
        w351 = "Calibrate" ("element")
        n176 = event-data() -> ()  [unwired: 1 in, 1 out]
        n177 = Enqueue Element(queue=w355, element=w351, error in (no error)=w354) -> (error out=w353:errorcluster)  [unwired: 1 in, 2 out]
        n178 = local write "P-State"(w351) -> ()
      }
      event #1 {
        w356 = "Switches" ("element")
        n179 = event-data() -> ()  [unwired: 1 in, 1 out]
        n180 = Enqueue Element(queue=w360, element=w356, error in (no error)=w359) -> (error out=w358:errorcluster)  [unwired: 1 in, 2 out]
        n181 = local write "P-State"(w356) -> ()
      }
      event #2 {
        w361 = "121 dB" ("element")
        n182 = event-data() -> ()  [unwired: 1 in, 1 out]
        n183 = Enqueue Element(queue=w365, element=w361, error in (no error)=w364) -> (error out=w363:errorcluster)  [unwired: 1 in, 2 out]
        n184 = local write "P-State"(w361) -> ()
      }
      event #3 {
        w366 = "70 dB" ("element")
        n185 = event-data() -> ()  [unwired: 1 in, 1 out]
        n186 = Enqueue Element(queue=w370, element=w366, error in (no error)=w369) -> (error out=w368:errorcluster)  [unwired: 1 in, 2 out]
        n187 = local write "P-State"(w366) -> ()
      }
      event #4 {
        w375 = "Configuration 1" ("element")
        n188 = event-data() -> ()  [unwired: 1 in, 3 out]
        n189 = Enqueue Element(queue=w374, element=w375, error in (no error)=w373) -> (error out=w372:errorcluster)  [unwired: 1 in, 2 out]
        n190 = local write "P-State"(w375) -> ()
      }
      event #5 {
        w381 = "Stop" ("element")
        n191 = event-data() -> ()  [unwired: 1 in, 1 out]
        n192 = Enqueue Element(queue=w378, element="Initialize", error in (no error)=w380) -> (queue out=w377:refnum<queue>, error out=w379:errorcluster)  [unwired: 1 in, 1 out]
        n193 = Enqueue Element(queue=w377, element=w381, error in (no error)=w379) -> (error out=w383:errorcluster)  [unwired: 1 in, 2 out]
        n194 = local write "P-State"(w381) -> ()
      }
      event #6 {
        n195 = event-data() -> ()  [unwired: 1 in, 1 out]
        n196 = Get Queue Status(queue=w388, error in (no error)=w384) -> (error out=w386:errorcluster)  [unwired: 1 in, 7 out]
        n197 = Unbundle By Name(w386) -> ("status"=w387:bool)
        "P-State" <- "Timeout" ("element")
      }
    }
  }
  "Instructions" <- "Noise Source Dummy Load calibration vi\n\n1 - Disable or turn off transmitter\n2 - Stow Antenna (point vertically)\n3 - Turn off all florescnt lights\n3 - Start the labview program by clicking the Run arrow\n     (left most button under  drop down menues)\n     start cycle time about 35 seconds\n4 - Wait for the red 'BUSY' light to change to green 'READY'\n     All the control buttons on the control panel are avtive.\n5 - Calibrate with the red  'Calibrate' button\n      calibration cycle time is about ? minutes\n6 - Exit the program with the red 'EXIT' button\n      exit cycle time about 20 seconds\n\nHints:\nWait for the green 'READY' light before clicking buttons\nAll the status leds on the 'Status' tab should be green during a calibration. " ("String")
